vi "ErrorHandling.Fglb.Check.vi"(8 "error in (no error)":errorcluster) -> (0 "error out":errorcluster, 2 "changed?":bool)   [LabVIEW 2016]
uses:
  CitTemplate/citTemplate.errData.ctl
  EventLog/EventLog.EventSource.ctl
  ErrorHandling.Fglb.Action.ctl
panel:
  out "Errors out":T1[](array[typedef])
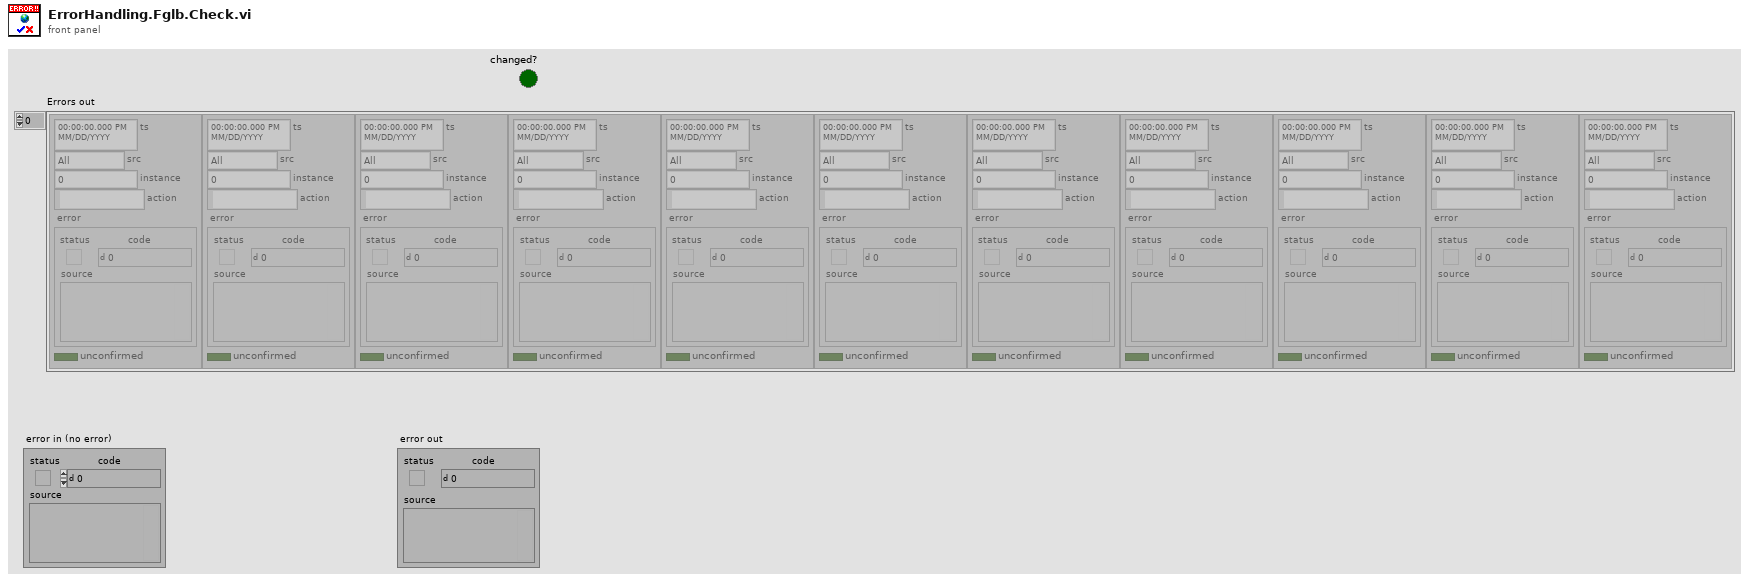
[diagram p1: front panel]
types:
  T1 = typedef "citTemplate.errData.ctl" = cluster{"ts":timestamp, "src":T2, "instance":i32, "action":string, "error":errorcluster, "unconfirmed":bool}
  T2 = typedef "EventLog.EventSource.ctl" = enum16{"All", "Gui", "Cache", "PLC1", "PLC2", "PLC3", "DB", "DB01", "DB02", "DB03", "DB04", "DB05", "DB06", "DB07", "DB08", "DB09", "DB10", "DB11", "DB12", "DB13", "DB14", "DB15", "DB16"}
  T3 = typedef "ErrorHandling.Fglb.Action.ctl" = enum16{"init", "add", "clear", "confirm", "check", "get"}
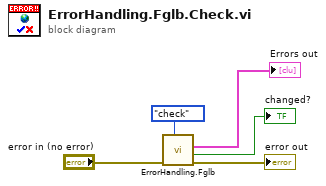
[diagram p0: block diagram]
diagram:
  n1 = call "ErrorHandling.Fglb.vi"("Action"=ErrorHandling.Fglb.Action."check", "error in (no error)"="error in (no error)") -> ("error out"=→"error out":errorcluster, "changed"=→"changed?":bool, "Errors out"=→"Errors out":T1[])  [unwired: 7 in]
